vi "createChildEvents.vi"(8 "error in (no error)":errorcluster, 11 "cameraSettingsEventManager in":refnum<class "cameraSettingsEventManager.lvclass">) -> (0 "error out":errorcluster, 3 "cameraSettingsEventManager out":refnum<class "cameraSettingsEventManager.lvclass">)   [LabVIEW 2011, in "Tools.lvlib" / "Settings.lvlib" / "cameraSettingsEventManager.lvclass"]
uses:
  cameraSettingsEventManager.lvclass
  cameraSettingsEventManager.lvclass/cameraSettingsEventManager.ctl
  Tools/Settings.lvlib
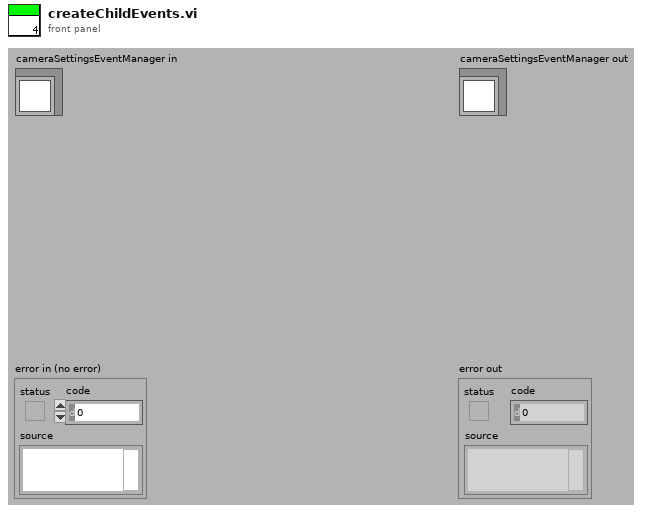
[diagram p1: front panel]
types:
  T1 = cluster{"loadCameraSettingsEvent":cluster{"cameraSettingFilePath":path}}
  T2 = cluster{"loadCameraSettingsEvent":refnum<user-event>}
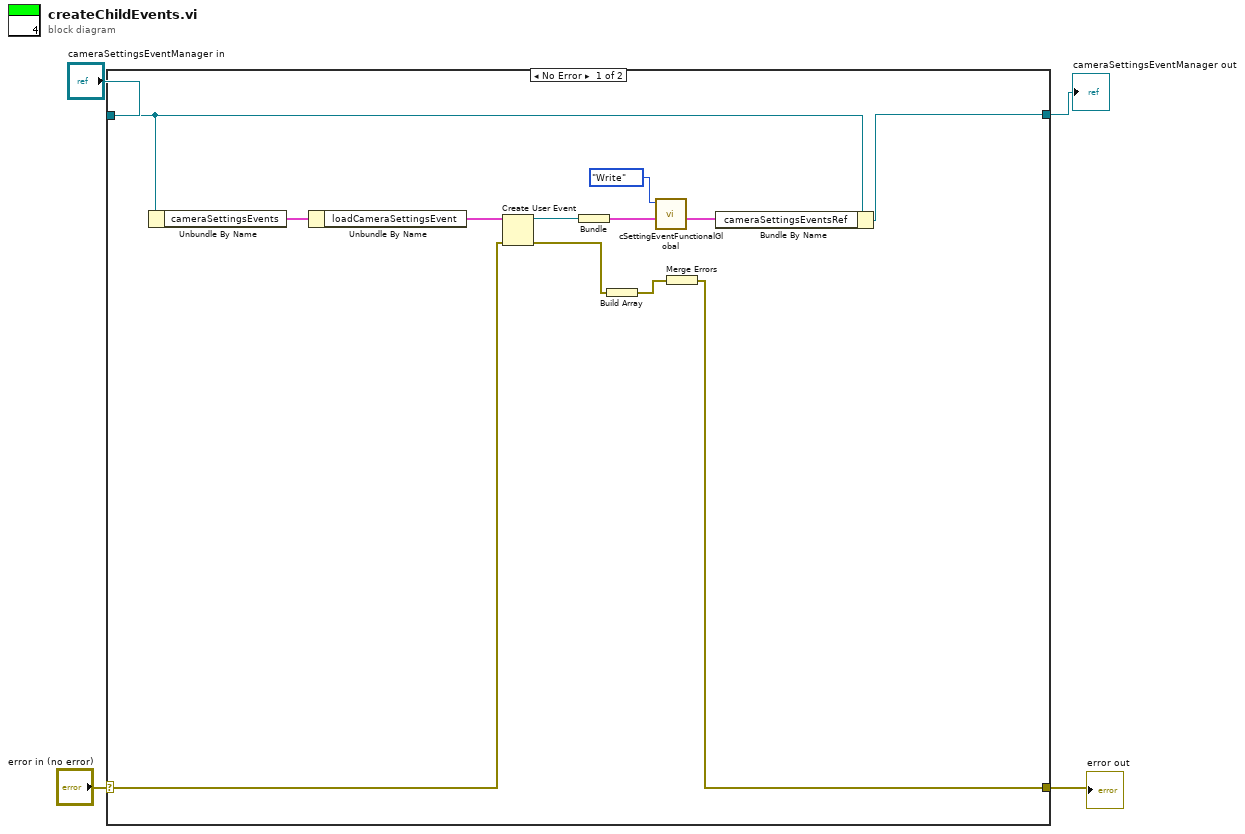
[diagram p0: block diagram]
diagram:
  n1 = case shown="No Error" "error in (no error)" {
    selector: "error in (no error)" -> [w6 w18]
    tunnel: "cameraSettingsEventManager in" -> [w8 w17]
    tunnel: [w7 w17] -> w2
    tunnel: [w5 w18] -> w1
    frame No Error {
      n2 = Unbundle By Name(w8) -> ("cameraSettingsEvents"=w16:T1)
      n3 = Unbundle By Name(w16) -> ("loadCameraSettingsEvent"=w15:cluster{"cameraSettingFilePath":path})
      n4 = Create User Event(user event datatype=w15, error in=w6) -> (user event=w14:refnum<user-event>, error out=w10:errorcluster)
      n5 = Bundle("loadCameraSettingsEvent"=w14) -> (w13:T2)  [unwired: 1 in]
      n6 = Build Array(w10) -> (w9:errorcluster[])
      n7 = call "cSettingEventFunctionalGlobal.vi"("cameraSettingsEventsRef"=w13, "Action"=enum16{"Write", "Read"}."Write") -> ("cameraSettingsEventsRef"=w11:T2)  [unwired: 9 in]
      n8 = Merge Errors(w9) -> (w5:errorcluster)
      n9 = Bundle By Name(cluster=w8, "cameraSettingsEventsRef"=w11) -> (w7:refnum<class "cameraSettingsEventManager.lvclass">)
    }
    frame Error {
    }
  }
  "error out" <- w1
  "cameraSettingsEventManager out" <- w2
